vi "load firmware.vi"(8 "error in (no error)":errorcluster, 9 "filename":string, 10 "store":bool, 11 "identifier":string) -> (0 "error out":errorcluster, 1 "filename out":string, 2 "function return":u32, 3 "identifier out":string)   [LabVIEW 2015, in "XGL_DPP.lvlib"]
doc: "EXTERN DECLSPEC unsigned int CALL_CONV load_firmware(char* identifier, bool store, char* filename);"
uses:
  XGL_DPP.lvlib
  D:/Scanning Software_Demokritos_2015_v6/libs/XGL_DPP.dll
panel:
  in  "board_num":u16
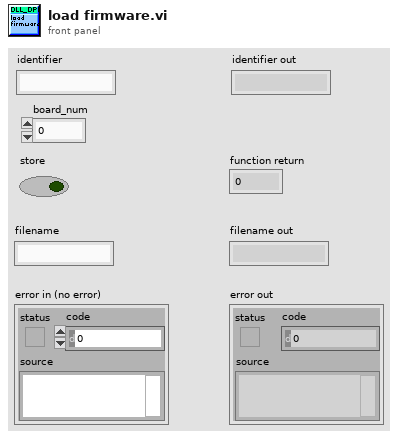
[diagram p1: front panel]
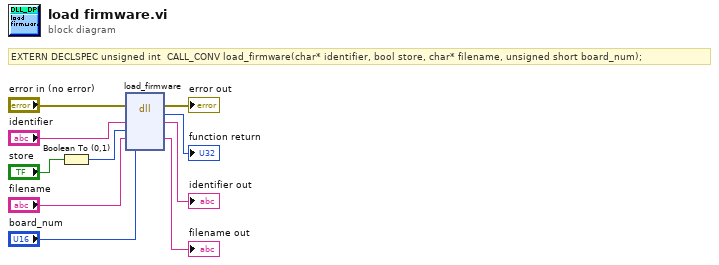
[diagram p0: block diagram]
diagram:
  # "EXTERN DECLSPEC unsigned int  CALL_CONV load_firmware(char* identifier, bool store, char* filename, unsigned short board_num);"
  n1 = Boolean To (0,1)(Boolean="store") -> (0, 1=w6:i16)
  n2 = dll-call lib="D:/Scanning Software_Demokritos_2015_v6/libs/XGL_DPP.*" fn="load_firmware"(error in="error in (no error)", "identifier"="identifier", "store"=w6, "filename"="filename", "board_num"="board_num") -> (error out=→"error out":errorcluster, "return type"=→"function return":u32, "identifier"=→"identifier out":string, "filename"=→"filename out":string)  [unwired: 4 in, 1 out]
